vi "CC Observation Calculate ABBA Dither Points.vi"(8 "error in (no error)":errorcluster, 10 "# Points":i32, 11 "B Offset":T5) -> (0 "error out":errorcluster, 3 "Dither":T2)   [LabVIEW 2024]
uses:
  typedefs/CC cluster RA and DEC.ctl
  typedefs/CC Dithering.ctl
  typedefs/CC cluster Offset Dithering.ctl
  typedefs/CC Dithering Offsets.ctl
  typedefs/CC enum Dither Selection.ctl
panel:
  in  "dither name":T1
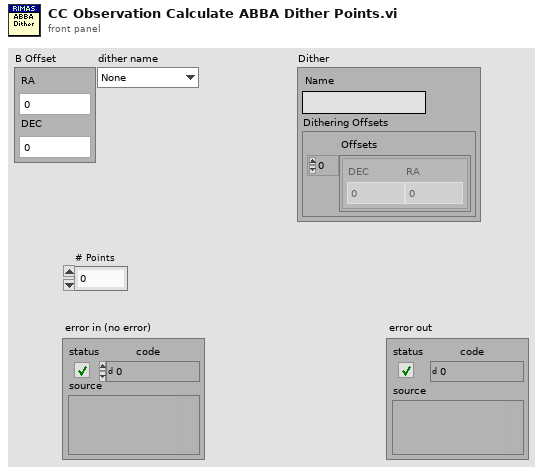
[diagram p1: front panel]
types:
  T1 = typedef "CC enum Dither Selection.ctl" = enum16{"None", "Circle", "Random", "ABBA", "OnOff"}
  T2 = typedef "CC Dithering.ctl" = cluster{"Name":string, "Dithering Offsets":T3}
  T3 = typedef "CC cluster Offset Dithering.ctl" = cluster{"Offsets":T4[]}
  T4 = typedef "CC Dithering Offsets.ctl" = cluster{"DEC":dbl, "RA":dbl}
  T5 = typedef "CC cluster RA and DEC.ctl" = cluster{"RA":dbl, "DEC":dbl}
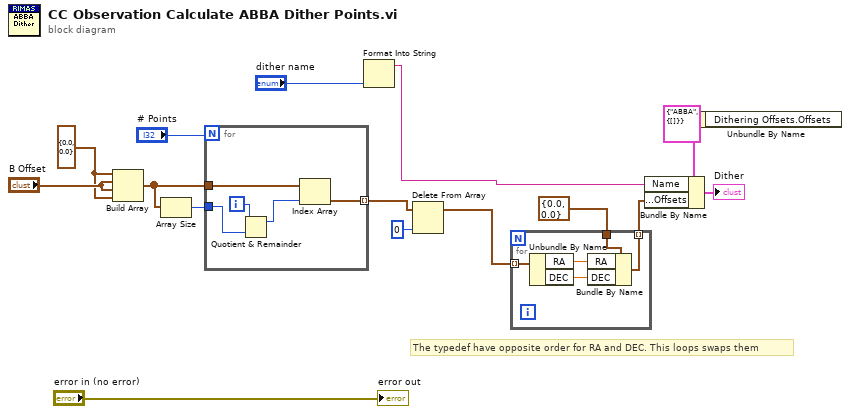
[diagram p0: block diagram]
diagram:
  w11 = T5 {"RA"=0.0, "DEC"=0.0} ("B Offset")
  w6 = T2 {"Name"="ABBA", "Dithering Offsets"={"Offsets"=[]}} ("Dithering Offsets")
  # "The typedef have opposite order for RA and DEC. This loops swaps them"
  n1 = Build Array(w11, "B Offset", "B Offset", w11) -> (w10:T5[])
  n2 = Array Size(array=w10) -> (size(s)=w9:i32)
  n3 = for {
    N: "# Points" -> [_]
    tunnel: w10 -> [w20]
    tunnel: w9 -> [w18]
    tunnel: [w16] -> w3 mode=indexing
    i -> [w19]
    n4 = Quotient & Remainder(x=w19, y=w18) -> (x-y*floor(x/y)=w17:i32)  [unwired: 1 out]
    n5 = Index Array(array=w20, index=w17) -> (element=w16:T5)
  }
  n6 = Format Into String("dither name") -> (resulting string=w7:string)  [unwired: 3 in, 1 out]
  n7 = Delete From Array(array=w3, index=0) -> (array with subset deleted=w1:T5[])  [unwired: 1 in, 1 out]
  n8 = for {
    tunnel: w1 -> [w23] mode=indexing
    tunnel: T4 {"DEC"=0.0, "RA"=0.0} ("Dither Offsets") -> [w24]
    tunnel: [w21] -> w4 mode=indexing
    n9 = Unbundle By Name(w23) -> ("RA"=w25:dbl, "DEC"=w22:dbl)
    n10 = Bundle By Name(cluster=w24, "RA"=w25, "DEC"=w22) -> (w21:T4)
  }
  n11 = Bundle By Name(cluster=w6, "Name"=w7, "Dithering Offsets.Offsets"=w4) -> (→"Dither":T2)
  n12 = Unbundle By Name(w6) -> ()  [unwired: 1 out]
  "error out" <- "error in (no error)"
